vi "XIPIN_Video_over_IP_FEC_Transmitter_1_0.vi"   [LabVIEW 2017]
doc: "The Xilinx, Inc. LogiCORE IP Video over IP FEC Transmitter is a broadcast application module that generates SMPTE 2022 Forward Error Correction redundant data from RTP encapsulated payload. It is capable of handling a large number of input streams and is suited for deploying in 1 Gb/s networks.\n------------------------------------\n<b>Need License</b> : Yes\n<b>Interface</b> : AXI4 AXI4-Stream"
uses:
  <vilib>/rvi/XilinxIP/XIPIN_XNode/niFpgaXIPIN.xnode
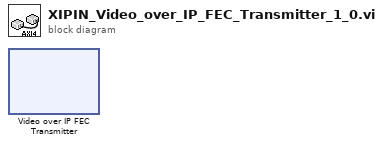
[diagram p0: block diagram]
diagram:
  n1 = xnode ("Video over IP FEC Transmitter")() -> ()
